vi "SVL Integration (N Ch).vi"(6 "reset filter (F)":bool, 7 "length units":i32(ring) items=["no change"=-1, "m"=0, "mm"=2, "microns"=3, "in"=1, "mils"=5], 8 "error in (no error)":errorcluster, 9 "highpass cutoff frequency":dbl=1.0 format="%.2f", 10 "integration type":T1(ring)=enum."double integration", 11 "scaled signals [EU]":waveform(dbl)[](array[waveform])) -> (0 "error out":errorcluster, 2 "unit labels":string[](array[string]), 3 "integrated signals":waveform(dbl)[](array[waveform]))   [LabVIEW 2017, in "SoundVib_Integration.lvlib"]
doc: "Converts acceleration to velocity or displacement using a time-domain waveform as the input. Wire data to the <B>scaled signal [EU]</B> input to determine the polymorphic instance to use or manually select the instance."
uses:
  <vilib>/addons/Sound and Vibration/svt_Integration/SoundVib_Integration.lvlib
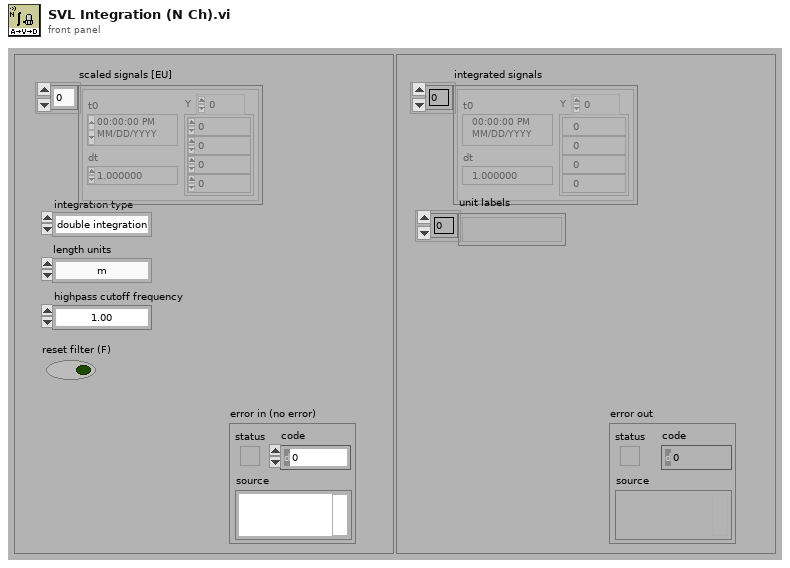
[diagram p1: front panel]
types:
  T1 = enum16{"single integration", "double integration"}
  T2 = cluster{"integration filter coefficients":cluster{"beta":dbl, "gamma":dbl, "alpha":dbl}, "highpass filter coefficients":cluster{"filter structure":enum32{"IIR 2nd Order", "IIR 4th Order"}, "Reverse Coefficients":dbl[], "Forward Coefficients":dbl[]}}
  T3 = cluster{"initial integration fiter state":cluster{"x(n-1) state":dbl, "y(n-1) state":dbl, "x(n-2) state":dbl, "y(n-2) state":dbl}, "initial highpass filter state":dbl[]}
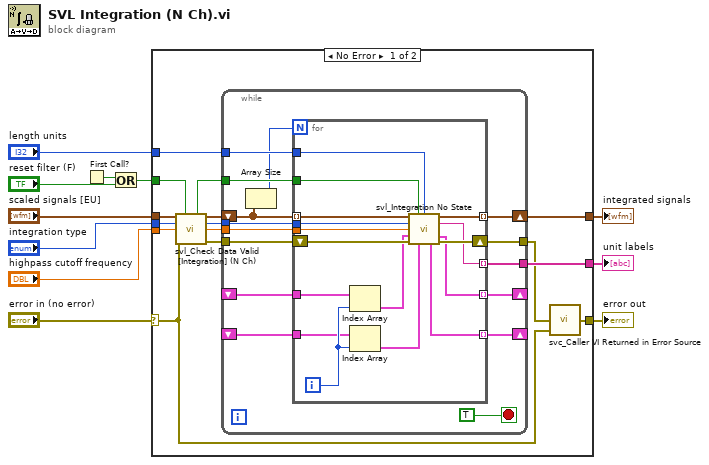
[diagram p0: block diagram]
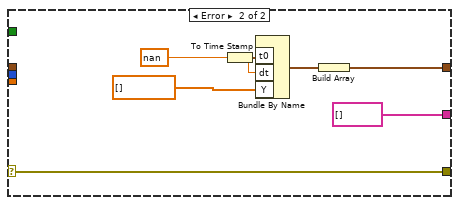
[diagram p2: hidden frame]
diagram:
  n1 = First Call?() -> (First Call?: T/F=w5:bool)
  n2 = Or(x=w5, y="reset filter (F)") -> (x .or. y?=w3:bool)
  n3 = case shown="No Error" "error in (no error)" {
    selector: "error in (no error)" -> [w12 w64]
    tunnel: "highpass cutoff frequency" -> [w15 _]
    tunnel: [w26 w59] -> w11
    tunnel: "scaled signals [EU]" -> [w20 _]
    tunnel: [w23 w64] -> w9
    tunnel: "length units" -> [w25 _]
    tunnel: [w24 string[] []] -> w7
    tunnel: w3 -> [w22 _]
    tunnel: "integration type" -> [w17 _]
    frame No Error {
      n4 = call <vilib>:"svl_Check Data Valid [Integration] (N Ch).vi"("scaled signals [EU]"=w20, "reset (in)"=w22, "integration type"=w17, "highpass cutoff frequency"=w15, "error in (no error)"=w12) -> ("reset (out)"=w21:bool, "integrated signals"=w19:waveform(dbl)[], "dup integration type"=w16:T1, "dup highpass cutoff frequency"=w14:dbl, "error out"=w18:errorcluster)  [unwired: 6 in]
      n5 = while {
        shift-left: _ -> [w29]
        shift-right: [w30] -> _
        tunnel: w21 -> [w31]
        tunnel: [w33] -> w24
        tunnel: w25 -> [w34]
        tunnel: [w36] -> w13
        tunnel: w18 -> [w37]
        tunnel: w16 -> [w38]
        tunnel: w14 -> [w40]
        shift-left: _ -> [w41]
        shift-right: [w27] -> _
        shift-right: [w39] -> w26
        shift-left: w19 -> [w32]
        stop <- TRUE stop-if-true
        n6 = Array Size(array=w32) -> (size(s)=w28:i32)
        n7 = for {
          N: w28 -> [_]
          tunnel: [w57] -> w39 mode=indexing
          shift-right: [w54] -> w36
          shift-left: w37 -> [w53]
          tunnel: w41 -> [w47]
          tunnel: w40 -> [w44]
          tunnel: w38 -> [w42]
          tunnel: w32 -> [w56] mode=indexing
          tunnel: w34 -> [w43]
          tunnel: [w50] -> w33 mode=indexing
          tunnel: w31 -> [w55]
          tunnel: [w45] -> w30 mode=indexing
          tunnel: w29 -> [w52]
          tunnel: [w48] -> w27 mode=indexing
          i -> [w51]
          n8 = Index Array(array=w52, index=w51) -> (element=w46:T2)
          n9 = Index Array(array=w47, index=w51) -> (element=w49:T3)
          n10 = call <vilib>:"svl_Integration No State.vi"("scaled signal [EU]"=w56, "reset filters"=w55, "length units"=w43, "integration type"=w42, "highpass cutoff frequency"=w44, "filter coefficents in"=w46, "error in (no error)"=w53, "initial filter state"=w49) -> ("scaled signal [EU]"=w57:waveform(dbl), "unit label"=w50:string, "filter coefficients out"=w45:T2, "final filter state"=w48:T3, "error out"=w54:errorcluster)  [unwired: 3 in]
        }
      }
      n11 = call <vilib>:"svc_Caller VI Returned in Error Source.vi"("warning input to caller"=w12, "error in (no error)"=w13) -> ("error out"=w23:errorcluster)  [unwired: 3 in]
    }
    frame Error {
      w62 = nan ("t0")
      n12 = To Time Stamp(1:w62) -> (0:w58:timestamp)
      n13 = Bundle By Name("t0"=w58, "dt"=w62, "Y"=dbl[] []) -> (w60:waveform(dbl))  [unwired: 1 in]
      n14 = Build Array(w60) -> (w59:waveform(dbl)[])
    }
  }
  "integrated signals" <- w11
  "error out" <- w9
  "unit labels" <- w7
